vi "file_renamer.vi"() -> ()   [LabVIEW 2010]
panel:
  in  "regular expression":string="LabVIEW 7.0 "
  in  "Replace match with:":string="Mano_Calib_"
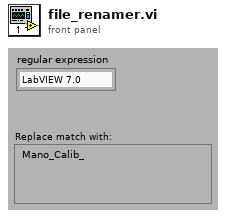
[diagram p1: front panel]
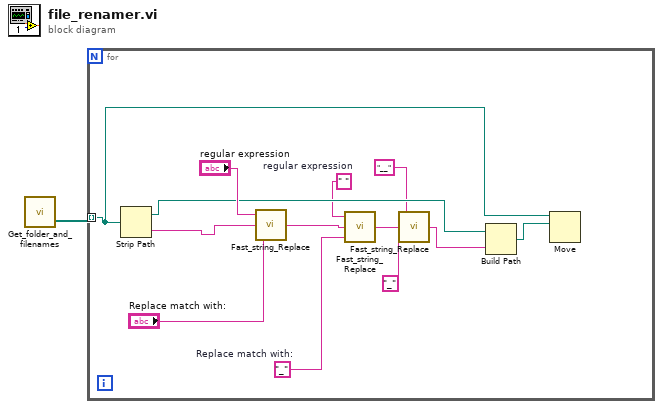
[diagram p0: block diagram]
diagram:
  n1 = call "Get_folder_and_filenames.vi"() -> ("Files"=w1:path[])  [unwired: 1 in, 1 out]
  n2 = for {
    tunnel: w1 -> [w11] mode=indexing
    w6 = "_"  # Replace match with:
    w7 = " "  # regular expression
    n3 = Strip Path(path=w11) -> (stripped path=w10:path, name=w14:string)
    n4 = call "Fast_string_Replace.vi"("Replace match with:"="Replace match with:", "Input String"=w14, "regular expression"="regular expression") -> ("Output String"=w8:string)  [unwired: 1 in, 1 out]
    n5 = call "Fast_string_Replace.vi"("Replace match with:"=w6, "Input String"=w8, "regular expression"=w7) -> ("Output String"=w3:string)  [unwired: 1 in, 1 out]
    n6 = call "Fast_string_Replace.vi"("Replace match with:"="_", "Input String"=w3, "regular expression"="__") -> ("Output String"=w2:string)  [unwired: 1 in, 1 out]
    n7 = Build Path(base path=w10, name or relative path=w2) -> (appended path=w9:path)
    n8 = Move(source path=w11, 10:w9) -> ()  [unwired: 3 in, 3 out]
  }
